vi "Get GUIDs from Constants VI.vi"(8 "error in":errorcluster, 11 "VI in":refnum<vi>) -> (0 "error out":errorcluster, 2 "set out":set{string}(c389), 3 "VI out":refnum<vi>)   [LabVIEW 2020, in "Utility.lvlib"]
uses:
  Utility.lvlib
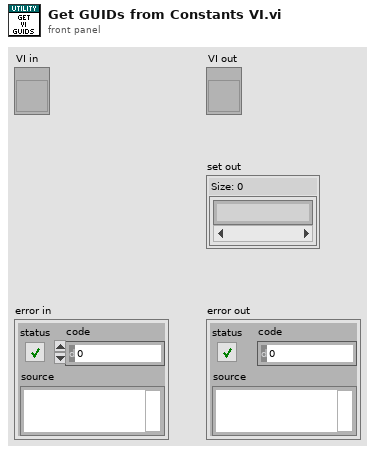
[diagram p1: front panel]
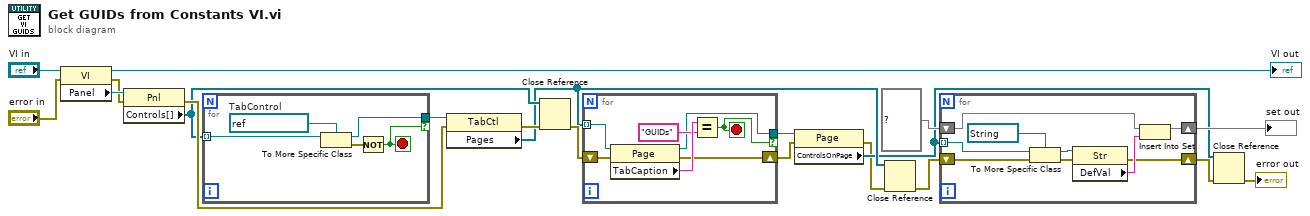
[diagram p0: block diagram]
diagram:
  n1 = property class="VI"(reference="VI in", error in="error in") -> (reference out=→"VI out":refnum<vi>, error out=w10:errorcluster, "Panel"=w16:refnum<vi>)
  n2 = property class="Pnl"(reference=w16, error in=w10) -> (error out=w9:errorcluster, "Controls[]"=w7:refnum<vi>[])  [unwired: 1 out]
  n3 = for {
    tunnel: w7 -> [w25] mode=indexing
    tunnel: [w23] -> w17 if=w21
    stop <- w21 stop-if-true
    w24 = refnum<vi> refnum  # TabControl
    n4 = To More Specific Class(target class=w24, reference=w25) -> (specific class reference=w23:refnum<vi>, error out=w22:errorcluster)  [unwired: 1 in]
    n5 = Not(x=w22) -> (.not. x?=w21:bool)
  }
  n6 = property class="TabCtl"(reference=w17, error in=w9) -> (error out=w12:errorcluster, "Pages"=w6:refnum<vi>[])  [unwired: 1 out]
  n7 = Close Reference(reference=w7, error in (no error)=w12) -> (error out=w8:errorcluster)
  n8 = for {
    tunnel: w6 -> [w32] mode=indexing
    tunnel: [w29] -> w18 if=w28
    shift-right: [w27] -> w3
    shift-left: w8 -> [w26]
    stop <- w28 stop-if-true
    n9 = property class="Page"(reference=w32, error in=w26) -> (reference out=w29:refnum<vi>, error out=w27:errorcluster, "TabCaption"=w31:string)
    n10 = Equal?(x=w31, y="GUIDs") -> (x = y?=w28:bool)
  }
  n11 = property class="Page"(reference=w18, error in=w3) -> (error out=w2:errorcluster, "ControlsOnPage"=w4:refnum<vi>[])  [unwired: 1 out]
  n12 = Close Reference(reference=w6, error in (no error)=w2) -> (error out=w1:errorcluster)
  n13 = for {
    tunnel: w4 -> [w41] mode=indexing
    shift-right: [w35] -> w20
    shift-left: set{string} {} ("set in") -> [w36]
    shift-right: [w34] -> w13
    shift-left: w1 -> [w33]
    n14 = To More Specific Class(target class=refnum<vi> refnum ("GUID.Import Frames"), reference=w41, error in=w33) -> (specific class reference=w39:refnum<vi>, error out=w38:errorcluster)
    n15 = property class="Str"(reference=w39, error in=w38) -> (error out=w34:errorcluster, "DefVal"=w37:string)  [unwired: 1 out]
    n16 = Insert Into Set(10:w37, 11:w36) -> (3:w35:set{string})  [unwired: 1 out]
  }
  "set out" <- w20
  n17 = Close Reference(reference=w4, error in (no error)=w13) -> (error out=→"error out":errorcluster)
